vi "Add cell to table.vi"(0 "PdfP Table":refnum<k24>, 1 "Row format with ref 2":T6, 2 "Image to Add [ ]":T7, 3 "Back Ground Color":u32(colorbox)=16777215, 5 "String":string, 7 "i":i32, 9 "Column Width (points)":dbl, 11 "error in (no error)":errorcluster, 12 "PDF Report IN":refnum<class "PDF Report Class.lvclass">) -> (4 "PdfP Table duplicate":refnum<k24>, 15 "error out":errorcluster)   [LabVIEW 2019]
doc: "Version 2.0\nDeveloped by Jean-Marc Simard\nCopyright © 2010, Exaprom Inc.\nAll rights reserved.\nLicense: BSD\n\nWith iTextSharp 4.1.6 (http://itextsharp.sourceforge.net)\nunder Mozilla Public License Version 1.1\n(http://www.mozilla.org/MPL/MPL-1.1.html)"
uses:
  C:/Program Files/National Instruments/LabVIEW 2019/user.lib/Exaprom PDF/DLL/itextsharp.dll
  DLL/itextsharp.dll
  <userlib>/Exaprom PDF/Controls/General Controls/Image to Add refnum [ ].ctl
  <userlib>/Exaprom PDF/Controls/Table Controls/Cell Cluster.ctl
  <userlib>/Exaprom PDF/Controls/Text Controls/Unicode/Type and run direction.ctl
  <userlib>/Exaprom PDF/Controls/Table Controls/Cell Alignment 20px.ctl
  <userlib>/Exaprom PDF/Controls/Table Controls/Text vertical arrangement.ctl
  <userlib>/Exaprom PDF/Controls/Font Controls/Font size.ctl
  <userlib>/Exaprom PDF/LV Class/PDF Report Class/PDF Report Class.lvclass
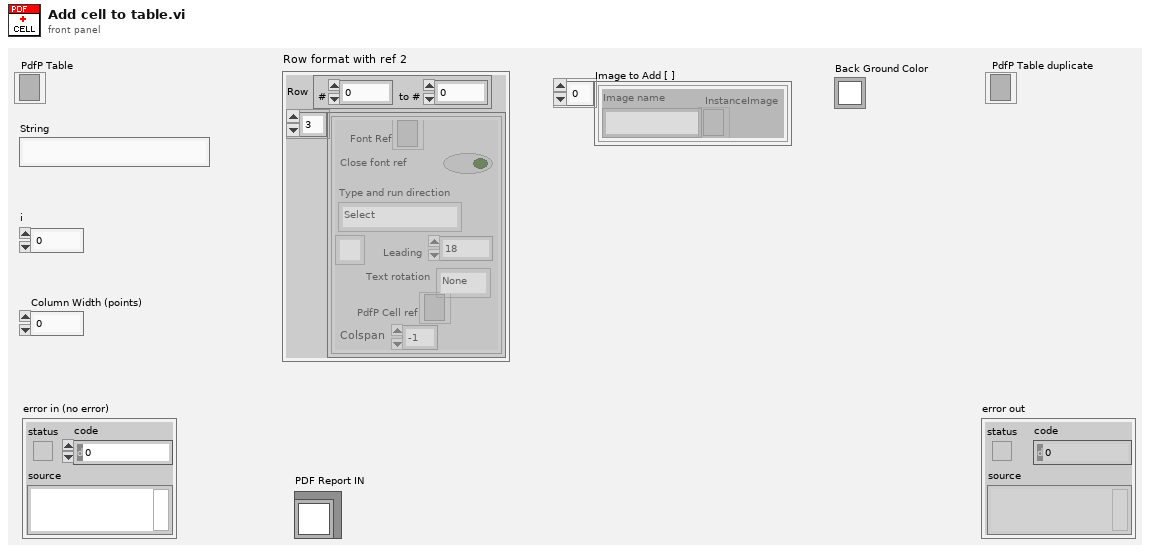
[diagram p1: front panel]
types:
  T1 = typedef "Cell Cluster.ctl" = cluster{"Font Ref":refnum<k24>, "Close font ref":bool, "Type and run direction":T2, "Cell Alignment":T3, "Text rotation":T4, "Leading":T5, "PdfP Cell ref":refnum<k24>, "Colspan":i8}
  T2 = typedef "Type and run direction.ctl" = enum16{"Select", "ASCII", "UTF-16", "UTF-16 (default)", "UTF-16 (LTR)", "UTF-16 (RTL)"}
  T3 = typedef "Cell Alignment 20px.ctl" = u16
  T4 = typedef "Text vertical arrangement.ctl" = enum16{"None", "Clockwise", "Counterclockwise"}
  T5 = typedef "Font size.ctl" = sgl
  T6 = cluster{"Row":cluster{"#":i16, "to #":i16}, "Cell [ ]":T1[]}
  T7 = typedef "Image to Add refnum [ ].ctl" = cluster{"Image name":string, "InstanceImage":refnum<k24>}[]
  T8 = typedef "Cell Vertical alignment.ctl" = enum16{"TOP", "MIDDLE", "BOTTOM"}
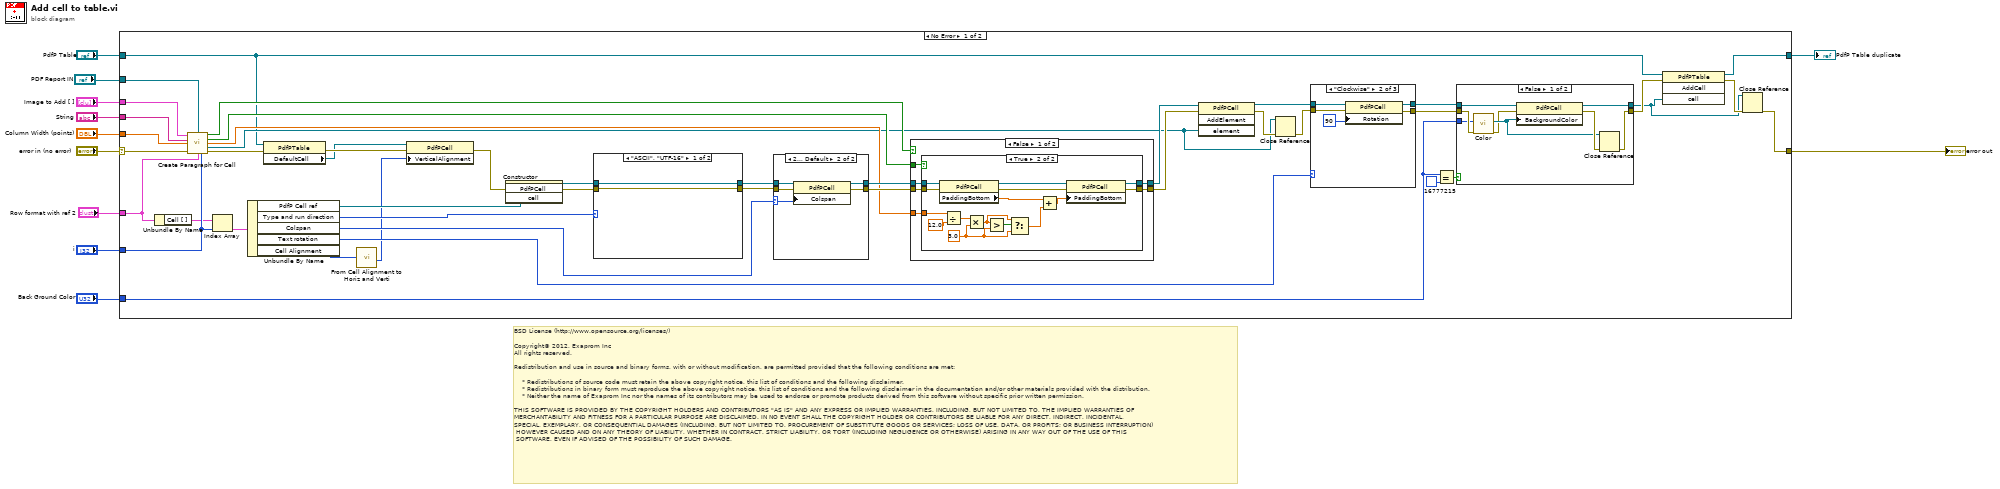
[diagram p0: block diagram]
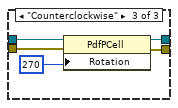
[diagram p3: hidden frame]
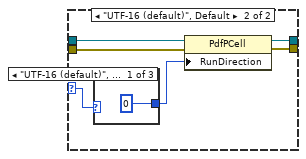
[diagram p4: hidden frame]
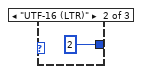
[diagram p5: hidden frame]
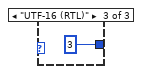
[diagram p6: hidden frame]
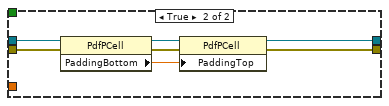
[diagram p9: hidden frame]
diagram:
  # "BSD License (http://www.opensource.org/licenses/)\n\nCopyright© 2012, Exaprom Inc\nAll rights reserved.\n\nRedistribution and use in source and binary forms, with or without modification, are permitted provided that the following conditions are met:\n\n    * Redistributions of source code must retain the above copyright notice, this list of conditions and the following disclaimer.\n    * Redistributions in binary form must reproduce the above copyright notice, this list of conditions and the following disclaimer in the documentation and/or other materials provided with the distribution.\n    * Neither the name of Exaprom Inc nor the names of its contributors may be used to endorse or promote products derived from this software without specific prior written permission.\n\nTHIS SOFTWARE IS PROVIDED BY THE COPYRIGHT HOLDERS AND CONTRIBUTORS \"AS IS\" AND ANY EXPRESS OR IMPLIED WARRANTIES, INCLUDING, BUT NOT LIMITED TO, THE IMPLIED WARRANTIES OF \nMERCHANTABILITY AND FITNESS FOR A PARTICULAR PURPOSE ARE DISCLAIMED. IN NO EVENT SHALL THE COPYRIGHT HOLDER OR CONTRIBUTORS BE LIABLE FOR ANY DIRECT, INDIRECT, INCIDENTAL,\nSPECIAL, EXEMPLARY, OR CONSEQUENTIAL DAMAGES (INCLUDING, BUT NOT LIMITED TO, PROCUREMENT OF SUBSTITUTE GOODS OR SERVICES; LOSS OF USE, DATA, OR PROFITS; OR BUSINESS INTERRUPTION)\n HOWEVER CAUSED AND ON ANY THEORY OF LIABILITY, WHETHER IN CONTRACT, STRICT LIABILITY, OR TORT (INCLUDING NEGLIGENCE OR OTHERWISE) ARISING IN ANY WAY OUT OF THE USE OF THIS\n SOFTWARE, EVEN IF ADVISED OF THE POSSIBILITY OF SUCH DAMAGE."
  n1 = case shown="No Error" "error in (no error)" {
    selector: "error in (no error)" -> [w34 w128]
    tunnel: [w50 w128] -> w2
    tunnel: [w19 w127] -> w10
    tunnel: "PdfP Table" -> [w17 w127]
    tunnel: "String" -> [w32 _]
    tunnel: "Image to Add [ ]" -> [w31 _]
    tunnel: "Column Width (points)" -> [w33 _]
    tunnel: "i" -> [w56 _]
    tunnel: "Back Ground Color" -> [w47 _]
    tunnel: "Row format with ref 2" -> [w30 _]
    tunnel: "PDF Report IN" -> [w22 _]
    frame No Error {
      n2 = Unbundle By Name(w30) -> ("Cell [ ]"=w46:T1[])
      n3 = call <userlib>:"Create Paragraph for Cell.vi"("Image to Add [ ]"=w31, "PDF Report IN"=w22, "String"=w32, "Column Width (points)"=w33, "error in (no error)"=w34, "Row format with ref"=w30, "i"=w56) -> ("Valid Image?"=w36:bool, "Modify Padding?"=w37:bool, "Font Size"=w38:sgl, "Paragraph refnum"=w35:refnum<k24>, "error out"=w18:errorcluster)  [unwired: 4 in]
      n4 = Index Array(array=w46, index=w56) -> (element=w39:T1)
      n5 = Unbundle By Name(w39) -> ("PdfP Cell ref"=w45:refnum<k24>, "Type and run direction"=w23:T2, "Colspan"=w29:i8, "Text rotation"=w24:T4, "Cell Alignment"=w21:T3)
      n6 = property class="PdfPTable"(reference=w17, error in=w18) -> (error out=w16:errorcluster, "DefaultCell"=w14:refnum<k24>)  [unwired: 1 out]
      n7 = call <userlib>:"From Cell Alignment to Horiz and Verti.vi"("Cell Alignment"=w21) -> ("Vertical Alignement"=w13:T8)  [unwired: 6 in, 1 out]
      n8 = property class="PdfPCell"(reference=w14, error in=w16, "VerticalAlignment"=w13) -> (error out=w15:errorcluster)  [unwired: 1 out]
      n9 = constructor class="PdfPCell"(error in=w15, "cell"=w45) -> (reference out=w20:refnum<k24>, error out=w42:errorcluster)  [unwired: 2 in, 2 out]
      n10 = case shown="\"ASCII\", \"UTF-16\"" w23 {
        selector: w23 -> [_ w72]
        tunnel: w20 -> [w70 w76]
        tunnel: w42 -> [w69 w75]
        tunnel: [w69 w74] -> w41
        tunnel: [w70 w73] -> w40
        frame "ASCII", "UTF-16" {
        }
        frame "UTF-16 (default)", Default {
          n11 = case shown="\"UTF-16 (default)\", Default" w72 {
            tunnel: [0 ("RunDirection") 2 ("RunDirection") 3 ("RunDirection")] -> w71
            frame "UTF-16 (default)", Default {
            }
            frame "UTF-16 (LTR)" {
            }
            frame "UTF-16 (RTL)" {
            }
          }
          n12 = property class="PdfPCell"(reference=w76, error in=w75, "RunDirection"=w71) -> (reference out=w73:refnum<k24>, error out=w74:errorcluster)
        }
      }
      n13 = case shown="2.., Default" w29 {
        selector: w29 -> [_ w82]
        tunnel: w40 -> [w81 w86]
        tunnel: w41 -> [w80 w85]
        tunnel: [w81 w84] -> w44
        tunnel: [w80 w83] -> w43
        frame 0, 1 {
        }
        frame 2.., Default {
          n14 = property class="PdfPCell"(reference=w86, error in=w85, "Colspan"=w82) -> (reference out=w84:refnum<k24>, error out=w83:errorcluster)
        }
      }
      n15 = case shown="False" w36 {
        tunnel: w43 -> [w89 w114]
        tunnel: [w88 w113] -> w49
        tunnel: w44 -> [w90 w112]
        tunnel: [w91 w110] -> w48
        tunnel: w37 -> [w92 _]
        tunnel: w38 -> [w87 _]
        frame False {
          n16 = case shown="True" w92 {
            tunnel: [w94 w107] -> w91
            tunnel: w90 -> [w94 w105]
            tunnel: w89 -> [w93 w104]
            tunnel: [w93 w106] -> w88
            tunnel: w87 -> [_ w101]
            frame False {
            }
            frame True {
              w96 = sgl 3.0 ("y")
              n17 = property class="PdfPCell"(reference=w105, error in=w104) -> (reference out=w108:refnum<k24>, error out=w109:errorcluster, "PaddingBottom"=w103:sgl)
              n18 = Divide(x=w101, y=sgl 12.0) -> (x/y=w99:sgl)
              n19 = Multiply(x=w99, y=w96) -> (x*y=w97:sgl)
              n20 = Greater?(x=w97, y=w96) -> (0:w98:bool)
              n21 = Select(t=w97, s=w98, f=w96) -> (s? t:f=w95:sgl)
              n22 = Add(x=w103, y=w95) -> (x+y=w102:sgl)
              n23 = property class="PdfPCell"(reference=w108, error in=w109, "PaddingBottom"=w102) -> (reference out=w107:refnum<k24>, error out=w106:errorcluster)
            }
          }
        }
        frame True {
          n24 = property class="PdfPCell"(reference=w112, error in=w114) -> (reference out=w111:refnum<k24>, error out=w115:errorcluster, "PaddingBottom"=w116:sgl)
          n25 = property class="PdfPCell"(reference=w111, error in=w115, "PaddingTop"=w116) -> (reference out=w110:refnum<k24>, error out=w113:errorcluster)
        }
      }
      n26 = invoke class="PdfPCell" method="AddElement"(reference=w48, error in=w49, "element"=w35) -> (reference out=w25:refnum<k24>, error out=w52:errorcluster)  [unwired: 1 in, 2 out]
      n27 = Close Reference(reference=w35, error in (no error)=w52) -> (error out=w26:errorcluster)
      n28 = case shown="\"Clockwise\"" w24 {
        tunnel: [w58 w63 w68] -> w28
        tunnel: [w57 w62 w67] -> w27
        tunnel: w26 -> [w57 w61 w66]
        tunnel: w25 -> [w58 w60 w65]
        frame "None", Default {
        }
        frame "Clockwise" {
          n29 = property class="PdfPCell"(reference=w60, error in=w61, "Rotation"=90) -> (reference out=w63:refnum<k24>, error out=w62:errorcluster)
        }
        frame "Counterclockwise" {
          n30 = property class="PdfPCell"(reference=w65, error in=w66, "Rotation"=270) -> (reference out=w68:refnum<k24>, error out=w67:errorcluster)
        }
      }
      n31 = Equal?(x=w47, y=u32 16777215 ("Color")) -> (x = y?=w54:bool)
      n32 = case shown="False" w54 {
        tunnel: w28 -> [w124 w126]
        tunnel: w27 -> [w119 w125]
        tunnel: [w123 w126] -> w12
        tunnel: [w121 w125] -> w53
        tunnel: w47 -> [w118 _]
        frame False {
          n33 = call <userlib>:"Color.vi"("error in (no error)"=w119, "Color"=w118) -> ("error out"=w117:errorcluster, "Color"=w120:refnum<k24>)  [unwired: 8 out]
          n34 = property class="PdfPCell"(reference=w124, error in=w117, "BackgroundColor"=w120) -> (reference out=w123:refnum<k24>, error out=w122:errorcluster)
          n35 = Close Reference(reference=w120, error in (no error)=w122) -> (error out=w121:errorcluster)
        }
        frame True {
        }
      }
      n36 = invoke class="PdfPTable" method="AddCell"(reference=w17, error in=w53, "cell"=w12) -> (reference out=w19:refnum<k24>, error out=w51:errorcluster)  [unwired: 1 in, 2 out]
      n37 = Close Reference(reference=w12, error in (no error)=w51) -> (error out=w50:errorcluster)
    }
    frame Error {
    }
  }
  "error out" <- w2
  "PdfP Table duplicate" <- w10
